vi "Setup.vi"() -> ()   [LabVIEW 2018]
uses:
  Global_Telescopio.vi
panel:
  in  "Case Constant\n(See Context Help) 2":bool
  in  "Case Constant\n(See Context Help)":bool
  out "Espelho#3":bool
  in  "Mover#3_COUDÉ":bool
  in  "Mover#3_CASS":bool
  out "PosSecundario":bool
  in  "Configuração":bool
  in  "ENGENHARIA":bool
  # "SETUP"
  # "Secundário para Foco"
  # "Conjunto Espelho #3"
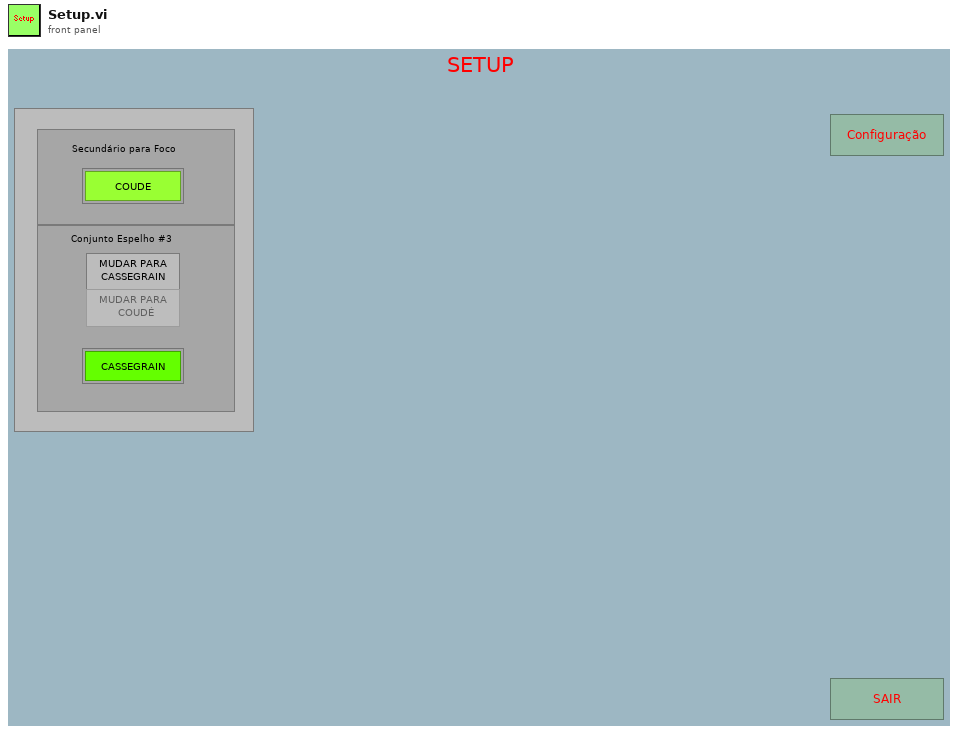
[diagram p1: front panel]
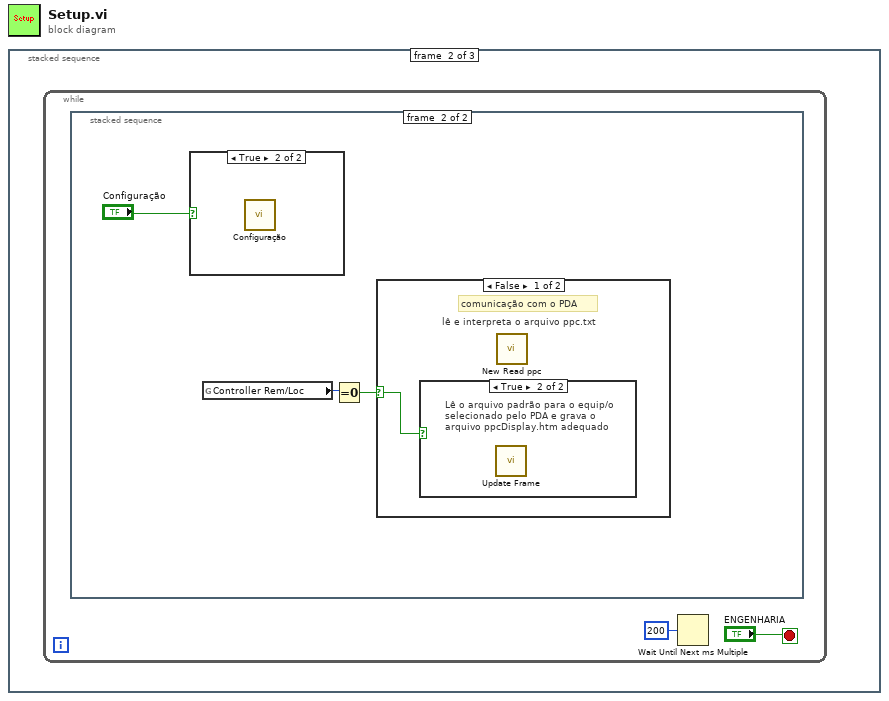
[diagram p0: block diagram]
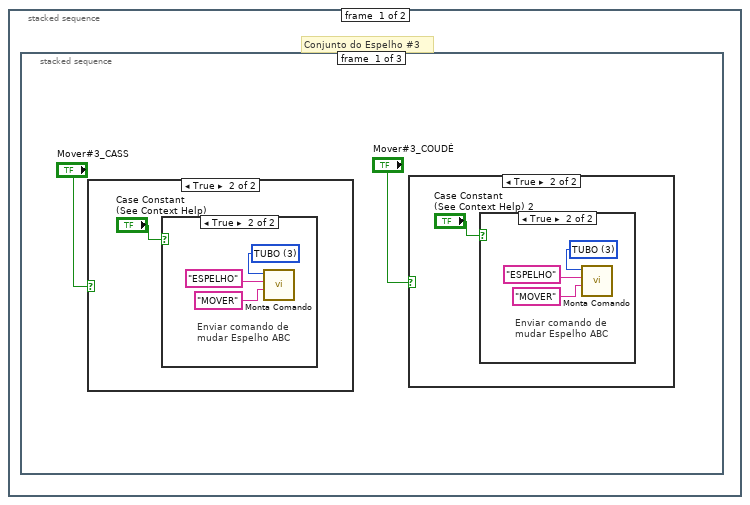
[diagram p3: hidden frame]
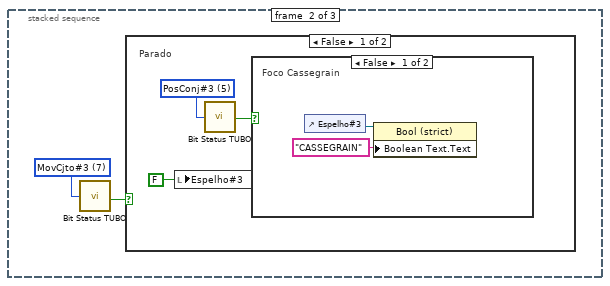
[diagram p8: hidden frame]
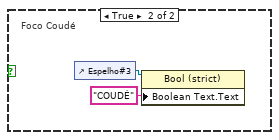
[diagram p9: hidden frame]
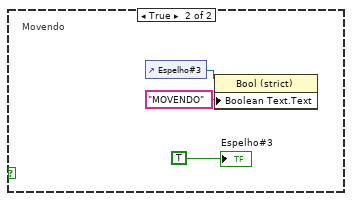
[diagram p10: hidden frame]
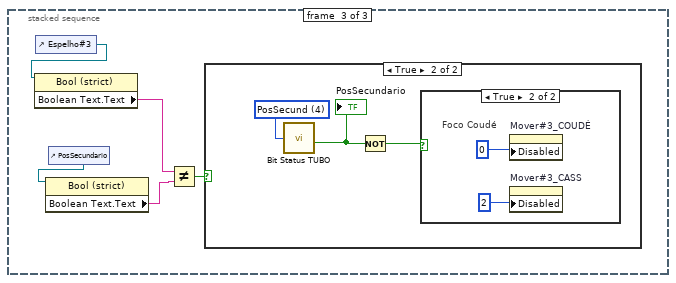
[diagram p11: hidden frame]
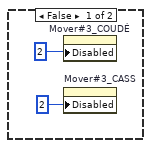
[diagram p12: hidden frame]
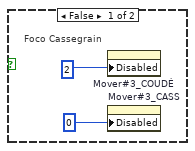
[diagram p13: hidden frame]
diagram:
  n1 = stacked-sequence {
    frame #0 {
      # "Inicialização"
    }
    frame #1 {
      n2 = while {
        stop <- "ENGENHARIA" stop-if-true
        n3 = stacked-sequence {
          frame #0 {
            # "Conjunto do Espelho #3"
            n4 = stacked-sequence {
              frame #0 {
                n5 = case shown="True" "Mover#3_CASS" {
                  frame False {
                  }
                  frame True {
                    n6 = case shown="True" "Case Constant\n(See Context Help)" {
                      frame False {
                      }
                      frame True {
                        w10 = u16 3 items=["ZERO", "AH", "DEC", "TUBO", "CUP"] ("Controlador")
                        # "Enviar comando de \nmudar Espelho ABC"
                        n7 = call "Monta Comando.vi"("Comando"="MOVER", "Dispositivo"="ESPELHO" ("Comando"), "Controlador"=w10) -> ()  [unwired: 3 in, 4 out]
                      }
                    }
                  }
                }
                n8 = case shown="True" "Mover#3_COUDÉ" {
                  frame False {
                  }
                  frame True {
                    n9 = case shown="True" "Case Constant\n(See Context Help) 2" {
                      frame False {
                      }
                      frame True {
                        w6 = u16 3 items=["ZERO", "AH", "DEC", "TUBO", "CUP"] ("Controlador")
                        # "Enviar comando de \nmudar Espelho ABC"
                        n10 = call "Monta Comando.vi"("Comando"="MOVER", "Dispositivo"="ESPELHO" ("Comando"), "Controlador"=w6) -> ()  [unwired: 3 in, 4 out]
                      }
                    }
                  }
                }
              }
              frame #1 {
                w14 = u16 7 items=["Alarme", "Atencao", "Erro", "Ocupado", "PosSecund", "PosConj#3", "MovFoco", "MovCjto#3", "Mov#4", "Mov#3", "Mov#2", "EspLamp", "HE", "NE", "EspLampRepouso", "EspLampCalibra"] ("NomeStatus")
                n11 = call "Bit Status TUBO.vi"("NomeStatus"=w14) -> ("StatBit"=w13:bool)
                n12 = case shown="False" w13 {
                  frame False {
                    w17 = u16 5 items=["Alarme", "Atencao", "Erro", "Ocupado", "PosSecund", "PosConj#3", "MovFoco", "MovCjto#3", "Mov#4", "Mov#3", "Mov#2", "EspLamp", "HE", "NE", "EspLampRepouso", "EspLampCalibra"] ("NomeStatus")
                    # "Parado"
                    n13 = local write "Espelho#3"(FALSE ("Espelho#3")) -> ()
                    n14 = call "Bit Status TUBO.vi"("NomeStatus"=w17) -> ("StatBit"=w16:bool)
                    n15 = case shown="False" w16 {
                      frame False {
                        # "Foco Cassegrain"
                        n16 = control-ref of="Espelho#3"() -> (w18:refnum<vi>)
                        n17 = property class="Bool (strict)"(reference=w18, "Boolean Text.Text"="CASSEGRAIN") -> ()  [unwired: 1 in, 2 out]
                      }
                      frame True {
                        # "Foco Coudé"
                        n18 = control-ref of="Espelho#3"() -> (w20:refnum<vi>)
                        n19 = property class="Bool (strict)"(reference=w20, "Boolean Text.Text"="COUDÉ") -> ()  [unwired: 1 in, 2 out]
                      }
                    }
                  }
                  frame True {
                    # "Movendo"
                    n20 = control-ref of="Espelho#3"() -> (w22:refnum<vi>)
                    n21 = property class="Bool (strict)"(reference=w22, "Boolean Text.Text"="MOVENDO") -> ()  [unwired: 1 in, 2 out]
                    "Espelho#3" <- TRUE ("Espelho#3")
                  }
                }
              }
              frame #2 {
                n22 = control-ref of="Espelho#3"() -> (w25:refnum<vi>)
                n23 = property class="Bool (strict)"(reference=w25) -> ("Boolean Text.Text"=w28:string)  [unwired: 1 in, 2 out]
                n24 = control-ref of="PosSecundario"() -> (w26:refnum<vi>)
                n25 = property class="Bool (strict)"(reference=w26) -> ("Boolean Text.Text"=w27:string)  [unwired: 1 in, 2 out]
                n26 = Not Equal?(x=w28, y=w27) -> (x != y?=w29:bool)
                n27 = case shown="True" w29 {
                  frame False {
                    n28 = property on="Mover#3_COUDÉ" class="Bool"("Disabled"=u8 2) -> ()  [unwired: 2 in, 2 out]
                    n29 = property on="Mover#3_CASS" class="Bool"("Disabled"=u8 2) -> ()  [unwired: 2 in, 2 out]
                  }
                  frame True {
                    w33 = u16 4 items=["Alarme", "Atencao", "Erro", "Ocupado", "PosSecund", "PosConj#3", "MovFoco", "MovCjto#3", "Mov#4", "Mov#3", "Mov#2", "EspLamp", "HE", "NE", "EspLampRepouso", "EspLampCalibra"] ("NomeStatus")
                    n30 = call "Bit Status TUBO.vi"("NomeStatus"=w33) -> ("StatBit"=w32:bool)
                    "PosSecundario" <- w32
                    n31 = Not(x=w32) -> (.not. x?=w34:bool)
                    n32 = case shown="True" w34 {
                      frame False {
                        # "Foco Cassegrain"
                        n33 = property on="Mover#3_COUDÉ" class="Bool"("Disabled"=u8 2) -> ()  [unwired: 2 in, 2 out]
                        n34 = property on="Mover#3_CASS" class="Bool"("Disabled"=u8 0) -> ()  [unwired: 2 in, 2 out]
                      }
                      frame True {
                        # "Foco Coudé"
                        n35 = property on="Mover#3_COUDÉ" class="Bool"("Disabled"=u8 0) -> ()  [unwired: 2 in, 2 out]
                        n36 = property on="Mover#3_CASS" class="Bool"("Disabled"=u8 2) -> ()  [unwired: 2 in, 2 out]
                      }
                    }
                  }
                }
              }
            }
          }
          frame #1 {
            n37 = case shown="True" "Configuração" {
              frame False {
              }
              frame True {
                n38 = call "Configuração.vi"() -> ()  [unwired: 1 in]
              }
            }
            n39 = global read "Global_Telescopio.vi" "Controller Rem/Loc"() -> (w40:i32)
            n40 = Equal To 0?(x=w40) -> (x = 0?=w39:bool)
            n41 = case shown="False" w39 {
              selector: w39 -> [w42 _]
              frame False {
                # "comunicação com o PDA"
                # "lê e interpreta o arquivo ppc.txt"
                n42 = case shown="True" w42 {
                  frame False {
                  }
                  frame True {
                    # "Lê o arquivo padrão para o equip/o\nselecionado pelo PDA e grava o\narquivo ppcDisplay.htm adequado"
                    n43 = call "Update Frame.vi"() -> ()  [unwired: 2 in, 4 out]
                  }
                }
                n44 = call "New Read ppc.vi"() -> ()  [unwired: 1 in]
              }
              frame True {
              }
            }
          }
        }
        n45 = Wait Until Next ms Multiple(millisecond multiple=u32 200) -> ()  [unwired: 1 out]
      }
    }
    frame #2 {
    }
  }
